vi "ScaleUp correction.vi"(8 "error in (no error)":errorcluster, 9 "Change?":bool, 10 "ScaleUp":dbl, 11 "Control-Client in":refnum<class "Control-Client.lvclass">) -> (0 "error out":errorcluster, 3 "Control-Client out":refnum<class "Control-Client.lvclass">)   [LabVIEW 2020, in "Control-Client.lvclass"]
uses:
  Control-Client.lvclass
  Control-Client.lvclass/Control-Client.ctl
  Experiments/Experiment.lvclass
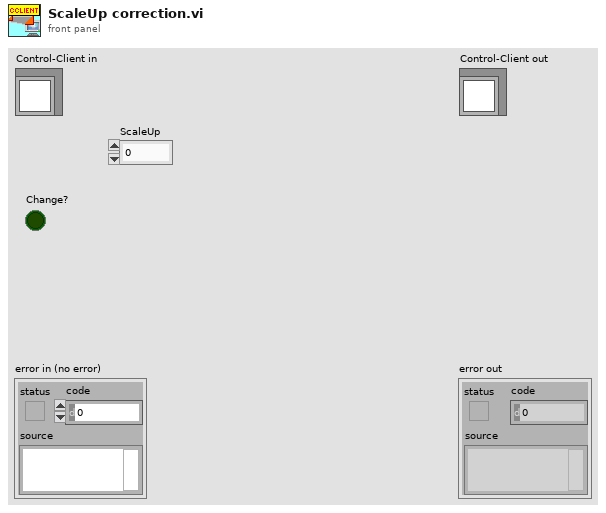
[diagram p1: front panel]
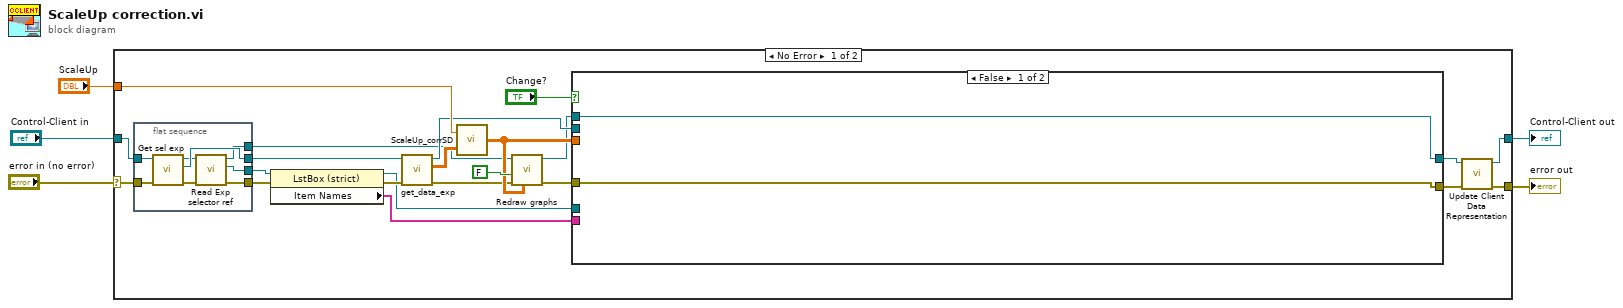
[diagram p0: block diagram]
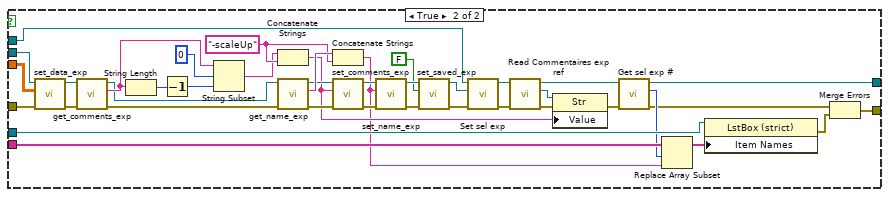
[diagram p2: hidden frame]
diagram:
  n1 = case shown="No Error" "error in (no error)" {
    selector: "error in (no error)" -> [w25 w79]
    tunnel: [w20 w79] -> w4
    tunnel: [w24 w78] -> w2
    tunnel: "Control-Client in" -> [w23 w78]
    tunnel: "ScaleUp" -> [w18 _]
    frame No Error {
      n2 = flat-sequence {
        tunnel: [w77] -> w26
        tunnel: w25 -> [w76]
        tunnel: w23 -> [w75]
        tunnel: [w74] -> w21
        tunnel: [w73] -> w19
        tunnel: [w70] -> w7
        frame #0 {
          n3 = call "Get sel exp.vi"("error in (no error)"=w76, "Control-Client in"=w75) -> ("error out"=w71:errorcluster, "Sel experiment"=w77:refnum<class "Experiment.lvclass">, "Control-Client out"=w72:refnum<class "Control-Client.lvclass">)  [unwired: 7 in]
          n4 = call "Read Exp selector ref.vi"("error in (no error)"=w71, "Control-Client in"=w72) -> ("error out"=w73:errorcluster, "Exp selector ref"=w74:refnum<vi>, "Control-Client out"=w70:refnum<class "Control-Client.lvclass">)  [unwired: 7 in]
        }
      }
      n5 = property on="Property Node" class="LstBox (strict)"(reference=w21, error in=w19) -> (reference out=w15:refnum<vi>, error out=w16:errorcluster, "Item Names"=w22:string[])
      n6 = call "get_data_exp.vi"("error in (no error)"=w16, "Experiment.lvclass in"=w26) -> ("error out"=w9:errorcluster, "Data"=w27:sgl[][], "Experiment.lvclass out"=w17:refnum<class "Experiment.lvclass">)  [unwired: 7 in]
      n7 = call "ScaleUp_corrSD.vi"("Data"=w27, "ScaleUp"=w18) -> ("Data corrected"=w11:dbl[][])
      n8 = call "Redraw graphs.vi"("Data"=w11, "error in (no error)"=w9, "Selected exp"=FALSE, "Control-Client in"=w7) -> ("error out"=w8:errorcluster, "Control-Client out"=w6:refnum<class "Control-Client.lvclass">)  [unwired: 6 in]
      n9 = case shown="False" "Change?" {
        tunnel: w22 -> [_ w54]
        tunnel: w8 -> [w28 w52]
        tunnel: w17 -> [_ w49]
        tunnel: w6 -> [w29 w46]
        tunnel: w15 -> [_ w45]
        tunnel: [w28 w38] -> w14
        tunnel: [w29 w37] -> w13
        tunnel: w11 -> [_ w32]
        frame False {
        }
        frame True {
          w62 = "-scaleUp" ("string")
          n10 = call "set_data_exp.vi"("error in (no error)"=w52, "Data"=w32, "Experiment.lvclass in"=w49) -> ("error out"=w50:errorcluster, "Experiment.lvclass out"=w51:refnum<class "Experiment.lvclass">)  [unwired: 7 in]
          n11 = call "get_comments_exp.vi"("error in (no error)"=w50, "Experiment.lvclass in"=w51) -> ("error out"=w68:errorcluster, "Comments"=w60:string, "Experiment.lvclass out"=w48:refnum<class "Experiment.lvclass">)  [unwired: 7 in]
          n12 = String Length(string=w60) -> (length=w58:i32)
          n13 = Decrement(x=w58) -> (x-1=w57:i32)
          n14 = String Subset(string=w60, offset (0)=0, length (rest)=w57) -> (substring=w56:string)
          n15 = Concatenate Strings(w56, w62) -> (w34:string)
          n16 = call "get_name_exp.vi"("error in (no error)"=w68, "Experiment.lvclass in"=w48) -> ("error out"=w69:errorcluster, "Exp name"=w67:string, "Experiment.lvclass out"=w47:refnum<class "Experiment.lvclass">)  [unwired: 7 in]
          n17 = Concatenate Strings(w67, w62) -> (w33:string)
          n18 = call "set_comments_exp.vi"("error in (no error)"=w69, "Comments"=w34, "Experiment.lvclass in"=w47) -> ("error out"=w65:errorcluster, "Experiment.lvclass out"=w66:refnum<class "Experiment.lvclass">)  [unwired: 7 in]
          n19 = call "set_name_exp.vi"("error in (no error)"=w65, "Exp name"=w33, "Experiment.lvclass in"=w66) -> ("error out"=w63:errorcluster, "Experiment.lvclass out"=w64:refnum<class "Experiment.lvclass">)  [unwired: 7 in]
          n20 = call "set_saved_exp.vi"("error in (no error)"=w63, "Saved"=FALSE, "Experiment.lvclass in"=w64) -> ("error out"=w55:errorcluster, "Experiment.lvclass out"=w53:refnum<class "Experiment.lvclass">)  [unwired: 7 in]
          n21 = call "Set sel exp.vi"("error in (no error)"=w55, "Experiment"=w53, "Control-Client in"=w46) -> ("error out"=w30:errorcluster, "Control-Client out"=w31:refnum<class "Control-Client.lvclass">)  [unwired: 7 in]
          n22 = call "Read Commentaires exp ref.vi"("error in (no error)"=w30, "Control-Client in"=w31) -> ("error out"=w41:errorcluster, "Commentaires exp ref"=w42:refnum<vi>, "Control-Client out"=w36:refnum<class "Control-Client.lvclass">)  [unwired: 7 in]
          n23 = property on="Property Node" class="Str"(reference=w42, error in=w41, "Value"=w34) -> (error out=w35:errorcluster)  [unwired: 1 out]
          n24 = call "Get sel exp #.vi"("error in (no error)"=w35, "Control-Client in"=w36) -> ("error out"=w39:errorcluster, "Exp sel #"=w43:i32, "Control-Client out"=w37:refnum<class "Control-Client.lvclass">)  [unwired: 7 in]
          n25 = Replace Array Subset(array=w54, new element=w33, index=w43) -> (w44:string[])
          n26 = property on="Property Node" class="LstBox (strict)"(reference=w45, "Item Names"=w44) -> (error out=w40:errorcluster)  [unwired: 1 in, 1 out]
          n27 = Merge Errors(w39, w40) -> (w38:errorcluster)
        }
      }
      n28 = call "Update Client Data Representation.vi"("error in (no error)"=w14, "Control-Client in"=w13) -> ("error out"=w20:errorcluster, "Control-Client out"=w24:refnum<class "Control-Client.lvclass">)  [unwired: 8 in]
    }
    frame Error {
    }
  }
  "error out" <- w4
  "Control-Client out" <- w2
